vi "2D Look-Up Table.vi"   [LabVIEW 2020, in "NI_AdvCtrl_nonlinear.lvlib"]
doc: "LabVIEW no longer supports this VI. You can obtain similar functionality by installing the LabVIEW Simulation Module.\n\nSearches for an element in a given 2D table that has a fractional x-index and y-index (interpolation)."
uses:
  <vilib>/addons/control/advanced/NI_AdvCtrl_nonlinear.lvlib
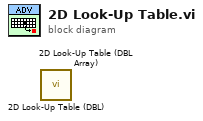
[diagram p0: block diagram]
diagram:
  n1 = call <vilib>:"2D Look-Up Table (DBL).vi"() -> ()  [unwired: 4 in, 1 out]
  n2 = call <vilib>:"2D Look-Up Table (DBL Array).vi"() -> ()  [unwired: 4 in, 1 out]
